vi "shutdown.vi"(8 "error in (no error)":errorcluster) -> (0 "error out":errorcluster)   [LabVIEW 2020, in "reqwest-labview.lvlib"]
doc: "Frees all stored response handles; call this once from your application's stop sequence after all requests are complete.\n\n\n\nvoid http_shutdown(void);"
uses:
  reqwest-labview.lvlib
  http_rs_labview.dll
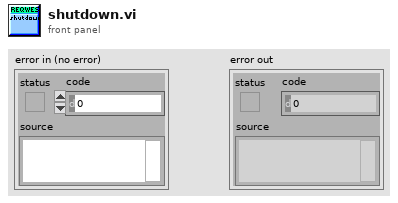
[diagram p1: front panel]
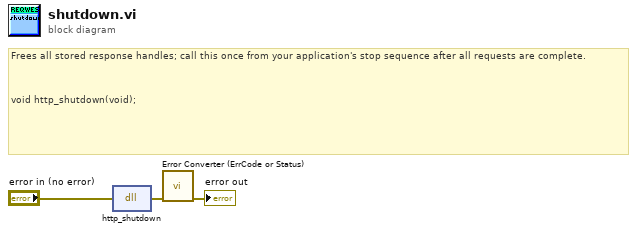
[diagram p0: block diagram]
diagram:
  # "Frees all stored response handles; call this once from your application's stop sequence after all requests are complete.\n\n\n\nvoid http_shutdown(void);"
  n1 = dll-call lib="C:/code/reqwest-labview/lv-src/shared-library/http_rs_labview.*" fn="http_shutdown"(error in="error in (no error)") -> (error out=w2:errorcluster)  [unwired: 3 in, 1 out]
  n2 = call "Error Converter (ErrCode or Status).vi"("error in (no error)"=w2) -> ("error out"=→"error out":errorcluster)  [unwired: 10 in]
